vi "step2 FindAndSolveBottomCornerPiece.vi"(8 "error in (no error)":errorcluster, 11 "cube in":T1) -> (0 "error out":errorcluster, 3 "cube out":T1)   [LabVIEW 2011]
doc: "Rotate cube as necessary so that the top middle piece matches the desired start colour.\n\nNo transformations are done in this VI, the operations are loaded on the the operation queue bus."
uses:
  Typedef/cube.ctl
  Typedef/face.ctl
  Typedef/operation.ctl
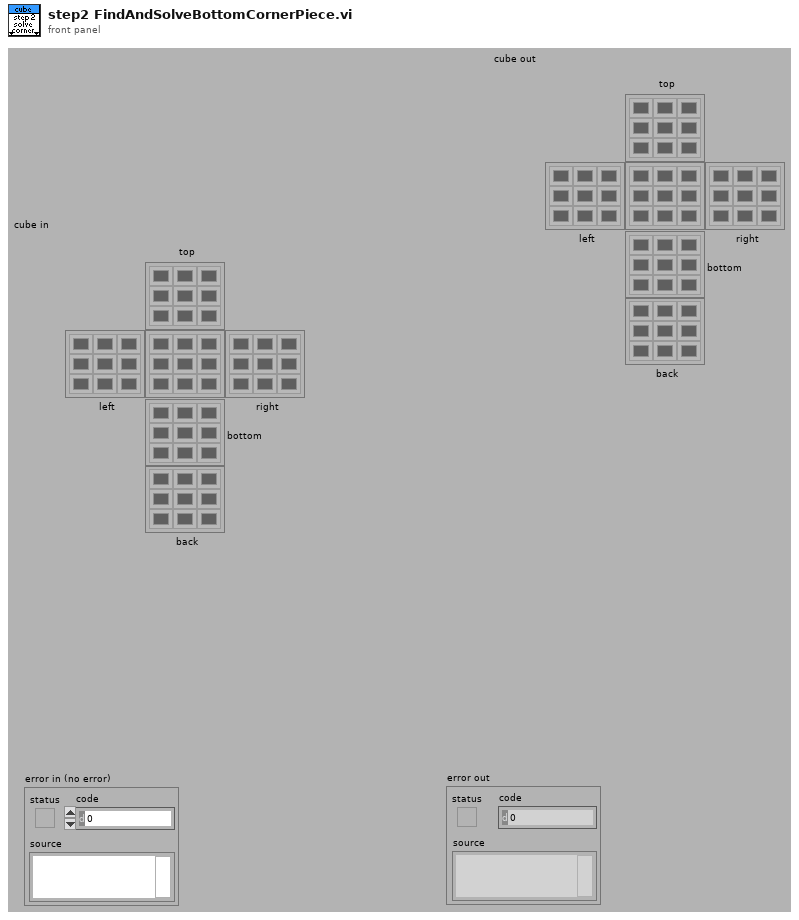
[diagram p1: front panel]
types:
  T1 = typedef "cube.ctl" = cluster{"top":T2, "left":T2, "right":T2, "bottom":T2, "back":T2, "front":T2}
  T2 = typedef "face.ctl" = u32[][]
  T3 = typedef "operation.ctl" = enum16{"nop", "T+", "T-", "F+", "F-", "L+", "L-", "R+", "R-", "B+", "B-", "<--", "-->", "^", "V"}
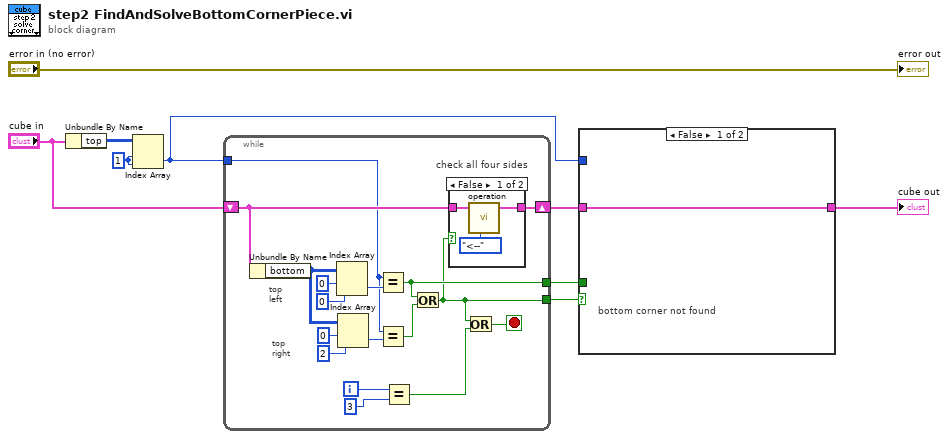
[diagram p0: block diagram]
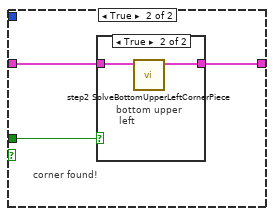
[diagram p3: hidden frame]
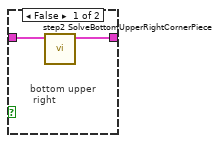
[diagram p4: hidden frame]
diagram:
  w7 = 1 ("index (row)")
  n1 = Unbundle By Name("cube in") -> ("top"=w8:T2)
  n2 = Index Array(array=w8, index (row)=w7, index (col)=w7) -> (element=w4:u32)
  n3 = while {
    tunnel: w4 -> [w17]
    shift-right: [w20] -> w1
    shift-left: "cube in" -> [w21]
    tunnel: [w14] -> w2
    tunnel: [w11] -> w3
    i -> [w23]
    stop <- w13 stop-if-true
    # "top\nright"
    # "top\nleft"
    # "check all four sides"
    n4 = Unbundle By Name(w21) -> ("bottom"=w15:T2)
    n5 = Index Array(array=w15, index (row)=0, index (col)=0 ("index (row)")) -> (element=w24:u32)
    n6 = Index Array(array=w15, index (row)=0, index (col)=2 ("index (row)")) -> (element=w16:u32)
    n7 = Equal?(x=w17, y=w24) -> (x = y?=w14:bool)
    n8 = Equal?(x=w17, y=w16) -> (x = y?=w10:bool)
    n9 = Equal?(x=w23, y=3 ("index (row)")) -> (x = y?=w12:bool)
    n10 = Or(x=w14, y=w10) -> (x .or. y?=w11:bool)
    n11 = case shown="False" w11 {
      tunnel: w21 -> [w28 w30]
      tunnel: [w27 w30] -> w20
      frame False {
        n12 = call "operation.vi"("operation"=operation."<--", "cube in"=w28) -> ("cube out"=w27:T1)  [unwired: 8 in, 1 out]
      }
      frame True {
      }
    }
    n13 = Or(x=w11, y=w12) -> (x .or. y?=w13:bool)
  }
  n14 = case shown="False" w3 {
    tunnel: w1 -> [w31 w33]
    tunnel: [w31 w32] -> w5
    tunnel: w4 -> [_ _]
    tunnel: w2 -> [_ w34]
    frame False {
      # "bottom corner not found"
    }
    frame True {
      # "corner found!"
      n15 = case shown="True" w34 {
        tunnel: w33 -> [w36 w38]
        tunnel: [w35 w37] -> w32
        frame False {
          # "bottom upper\n right"
          n16 = call "step2 SolveBottomUpperRightCornerPiece.vi"("cube in"=w36) -> ("cube out"=w35:T1)  [unwired: 9 in, 1 out]
        }
        frame True {
          # "bottom upper\n left"
          n17 = call "step2 SolveBottomUpperLeftCornerPiece.vi"("cube in"=w38) -> ("cube out"=w37:T1)  [unwired: 9 in, 1 out]
        }
      }
    }
  }
  "cube out" <- w5
  "error out" <- "error in (no error)"
